vi "Digital Channels--constant.vi"() -> (3 "Digital Channels--constant":tag[](array[tag])=["A/DIO0", "A/DIO1", "A/DIO2", "A/DIO3", "A/DIO4", "A/DIO5", "A/DIO6", "A/DIO7", "A/DIO8", "A/DIO9", "A/DIO10", "A/DIO10", "A/DIO12", "A/DIO13", "A/DIO14", "A/DIO15"])   [LabVIEW 2021, in "Common Files.lvlib"]
uses:
  Common Files.lvlib
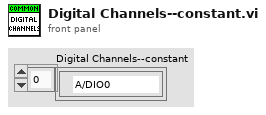
[diagram p1: front panel]
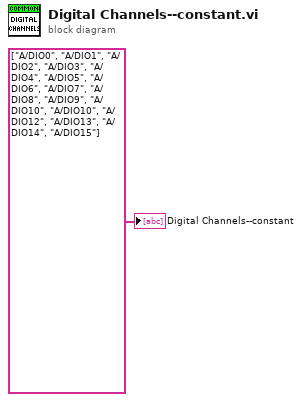
[diagram p0: block diagram]
diagram:
  "Digital Channels--constant" <- tag[] ["A/DIO0", "A/DIO1", "A/DIO2", "A/DIO3", "A/DIO4", "A/DIO5", "A/DIO6", "A/DIO7", "A/DIO8", "A/DIO9", "A/DIO10", "A/DIO10", "A/DIO12", "A/DIO13", "A/DIO14", "A/DIO15"] ("Channel Names")
